vi "TX_CamAcqModule.vi"(8 "error out":errorcluster, 10 "Event Registration Refnum":refnum<event-registration>, 11 "queue out":refnum<queue>) -> (0 "error out 2":errorcluster, 3 "queue out 2":refnum<queue>)   [LabVIEW 2023]
uses:
  TX_Control 3.ctl
  <vilib>/userDefined/High Color/IMAQdx.ctl
  <vilib>/vision/Image Controls.llb/IMAQ Image.ctl
  <vilib>/vision/driver/NI_Vision_Acquisition_Software.lvlib
  TX_Cluster1TypeDef.ctl
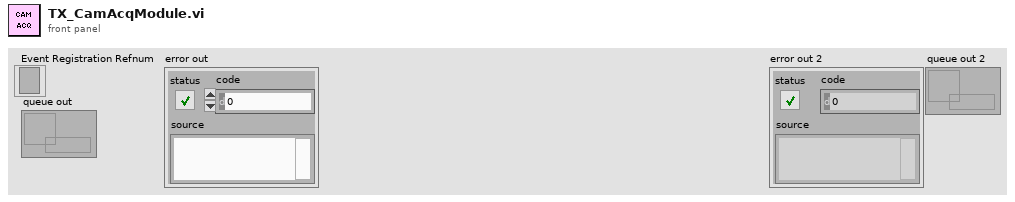
[diagram p1: front panel]
types:
  T1 = typedef "TX_Cluster1TypeDef.ctl" = cluster{"Enum":T2, "CamSel":variant, "CamView":variant}
  T2 = typedef "TX_Control 3.ctl" = enum16{"Default", "PathLoaded", "StartCamera", "TakePhoto", "EnableTCP", "Cam2Display", "CloseAll"}
  T3 = typedef "IMAQ Image.ctl" = refnum<image>
  T4 = typedef "IMAQdx.ctl" = refnum<k21>
  T5 = typedef "Image Type" = u32
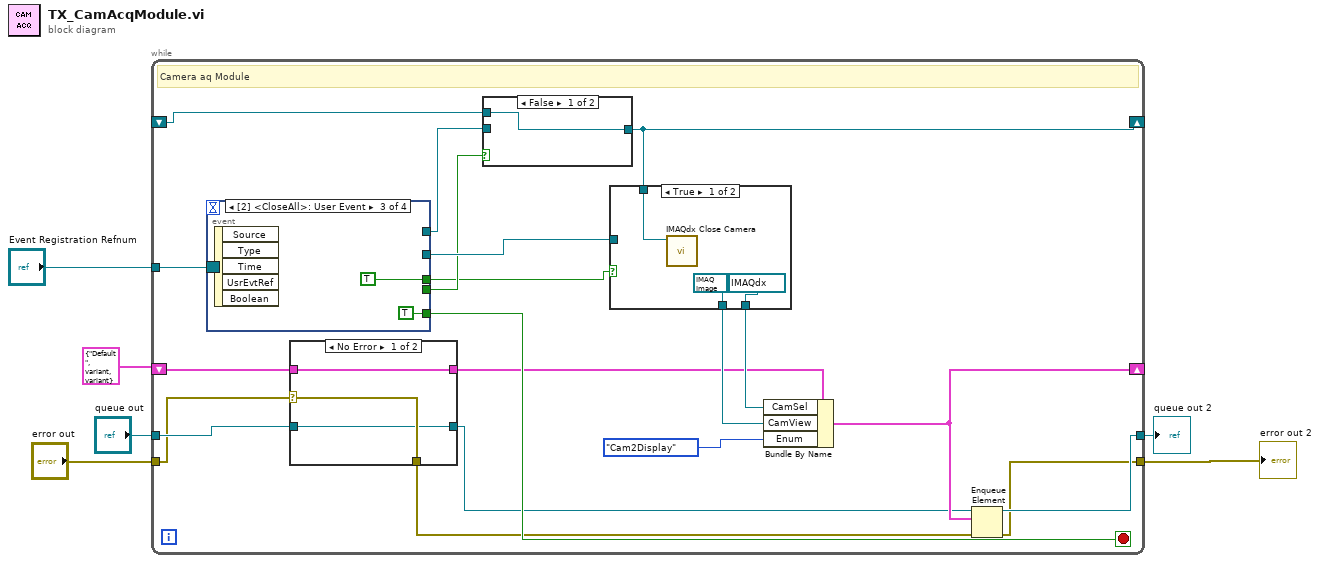
[diagram p0: block diagram]
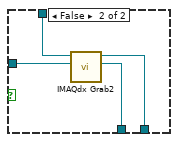
[diagram p2: hidden frame]
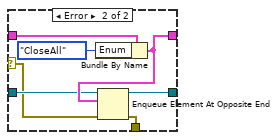
[diagram p3: hidden frame]
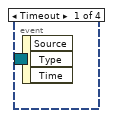
[diagram p5: hidden frame]
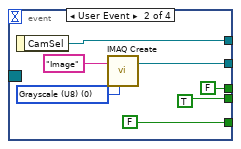
[diagram p6: hidden frame]
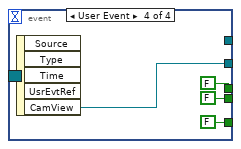
[diagram p7: hidden frame]
diagram:
  n1 = while {
    shift-right: [w25] -> _
    shift-left: T1 {"Enum"=enum."Default", "CamSel"=variant(refnum<image> refnum), "CamView"=variant(refnum<image> refnum)} ("Cluster") -> [w13]
    tunnel: [w24] -> w1
    tunnel: "queue out" -> [w11]
    tunnel: "error out" -> [w9]
    tunnel: [w23] -> w2
    tunnel: "Event Registration Refnum" -> [w22]
    shift-right: [w17] -> _
    shift-left: _ -> [w16]
    stop <- w26 stop-if-true
    # "Camera aq Module"
    n2 = event shown="[2] <CloseAll>: User Event" {
      selector: w22 -> [_ _ _ _]
      dyn-events: _ -> [_ _ _ _]
      timeout: _ -> [_ _ _ _]
      tunnel: [_ FALSE TRUE FALSE] -> w26
      tunnel: [_ w50 _ _] -> w18
      tunnel: [_ w49 _ w58] -> w20
      tunnel: [_ TRUE _ FALSE] -> w19
      tunnel: [_ FALSE TRUE FALSE] -> w7
      event Timeout {
        n3 = event-data() -> ()  [unwired: 1 in, 3 out]
      }
      event User Event {
        w47 = T5 0 items=["Grayscale (U8)", "Grayscale (I16)", "Grayscale (SGL)", "Complex (CSG)", "RGB (U32)", "HSL (U32)", "RGB (U64)", "Grayscale (U16)"] ("Image Type")
        n4 = event-data() -> ("CamSel"=w50:T4)  [unwired: 1 in]
        n5 = call "IMAQ Create"("Image Name"="Image", "Image Type"=w47) -> ("New Image"=w49:T3)  [unwired: 3 in, 1 out]
      }
      event User Event {
        n6 = event-data() -> ()  [unwired: 1 in, 5 out]
      }
      event User Event {
        n7 = event-data() -> ("CamView"=w58:T3)  [unwired: 1 in, 4 out]
      }
    }
    n8 = case shown="No Error" w9 {
      selector: w9 -> [w35 w39]
      tunnel: [w36 w41] -> w12
      tunnel: w13 -> [w36 w43]
      tunnel: w11 -> [w34 w40]
      tunnel: [w35 w38] -> w8
      tunnel: [w34 w37] -> w10
      frame No Error {
      }
      frame Error {
        n9 = Bundle By Name(cluster=w43, "Enum"=TX_Control_3."CloseAll") -> (w41:T1)
        n10 = Enqueue Element At Opposite End(queue=w40, element=w41, error in (no error)=w39) -> (queue out=w37:refnum<queue>, error out=w38:errorcluster)  [unwired: 1 in, 1 out]
      }
    }
    n11 = case shown="False" w19 {
      tunnel: w18 -> [_ w45]
      tunnel: [w44 w45] -> w17
      tunnel: w16 -> [w44 _]
      frame False {
      }
      frame True {
      }
    }
    n12 = case shown="True" w7 {
      tunnel: w20 -> [_ w33]
      tunnel: w17 -> [w27 w32]
      tunnel: [T3 refnum ("Image Out") w31] -> w15
      tunnel: [T4 "cam0" ("Session Out") w30] -> w14
      frame True {
        n13 = call <vilib>:"IMAQdx Close Camera.vi"("Session In"=w27) -> ()  [unwired: 10 in, 1 out]
      }
      frame False {
        n14 = call <vilib>:"IMAQdx Grab2.vi"("Image In"=w33, "Session In"=w32) -> ("Image Out"=w31:T3, "Session Out"=w30:T4)  [unwired: 6 in, 2 out]
      }
    }
    n15 = Bundle By Name(cluster=w12, "CamSel"=w14, "CamView"=w15, "Enum"=TX_Control_3."Cam2Display") -> (w25:T1)
    n16 = Enqueue Element(queue=w10, element=w25, error in (no error)=w8) -> (queue out=w24:refnum<queue>, error out=w23:errorcluster)  [unwired: 1 in, 1 out]
  }
  "error out 2" <- w2
  "queue out 2" <- w1
